vi "process_hit.vi"(7 "hammerIndex":i32, 11 "config":T1={"rate"=1652.0, "duration"=1.0, "thr"=100.0, "preTrigger"=100.0, "cutoff"=-3.0, "Filtro"=enum."Desativado", "highPass"=1000.0, "lowPass"=1000.0, "updateTime"=50.0} {"updateTime" format="%#_g ms"; "lowPass" format="%#_g Hz"; "highPass" format="%#_g Hz"; "cutoff" format="%#_g dB"; "preTrigger" format="%#_g ms"; "thr" format="%#_g N"; "duration" format="%#_g s"; "rate" min=1652.0 max=51200.0 format="%#_g Hz"}) -> ()   [LabVIEW 2016]
uses:
  MainFGV/Settings/Advanced/AdvancedConfig.ctl
  MainFGV/MainFGV_mods.ctl
panel:
  out "error out":errorcluster
  in  "error in":errorcluster
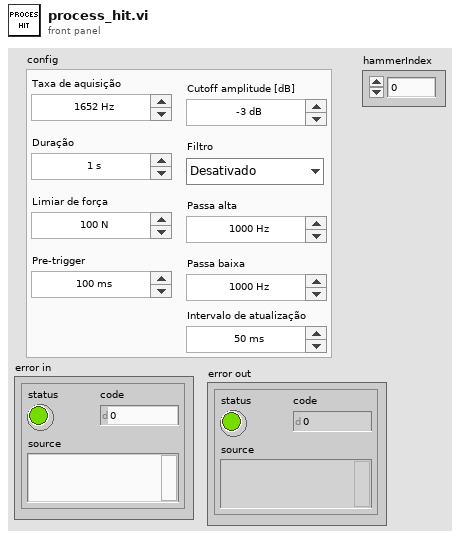
[diagram p1: front panel]
types:
  T1 = typedef "AdvancedConfig.ctl" = cluster{"rate":dbl, "duration":dbl, "thr":dbl, "preTrigger":dbl, "cutoff":dbl, "Filtro":enum16{"Desativado", "Passa banda", "Passa alta", "Passa baixa"}, "highPass":dbl, "lowPass":dbl, "updateTime":dbl}
  T2 = typedef "MainFGV_mods.ctl" = enum16{"Init", "Config", "Advanced", "CreateTask", "Register", "Start", "Record", "End"}
  T3 = typedef "results_data.ctl" = cluster{"config":T1, "hammer":waveform(dbl), "acelerometers":waveform(dbl)[], "hammerIndex":i32}
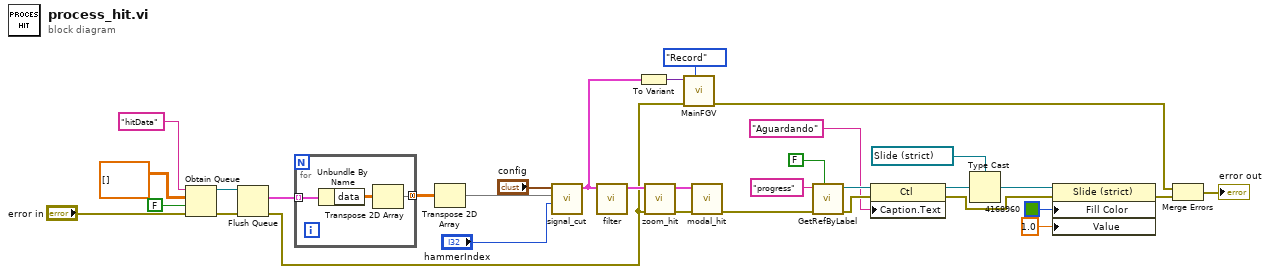
[diagram p0: block diagram]
diagram:
  n1 = Obtain Queue(name (unnamed)="hitData", element data type=dbl[][] [] ("data"), create if not found? (T)=FALSE, error in (no error)="error in") -> (queue out=w10:refnum<queue>, error out=w11:errorcluster)  [unwired: 1 in, 1 out]
  n2 = Flush Queue(queue=w10, error in (no error)=w11) -> (remaining elements=w9:cluster{"data":dbl[][]}[], error out=w5:errorcluster)  [unwired: 1 out]
  n3 = for {
    tunnel: w9 -> [w36] mode=indexing
    tunnel: [w34] -> w8 mode=concatenating
    n4 = Unbundle By Name(w36) -> ("data"=w35:dbl[][])
    n5 = Transpose 2D Array(2D array=w35) -> (transposed array=w34:dbl[][])
  }
  n6 = Transpose 2D Array(2D array=w8) -> (transposed array=w29:dbl[][])
  n7 = call "signal_cut.vi"("hammerIndex"="hammerIndex", "data"=w29, "config"="config") -> ("data_out"=w6:T3)  [unwired: 8 in]
  n8 = call "filter.vi"("data_in"=w6) -> ("data_out"=w30:T3)  [unwired: 10 in]
  n9 = To Variant(anything=w6) -> (Variant=w4:variant)
  n10 = call "zoom_hit.vi"("error in"=w5, "data_in"=w30) -> ("error out"=w17:errorcluster, "data_out"=w16:T3)  [unwired: 8 in]
  n11 = call "MainFGV.vi"("FGV_mods"=MainFGV_mods."Record", "Error In"=w5, "DataIn"=w4) -> ("Error Out"=w2:errorcluster)  [unwired: 7 in, 1 out]
  n12 = call "modal_hit.vi"("error in"=w17, "data_in"=w16) -> ("error out"=w15:errorcluster)  [unwired: 8 in, 1 out]
  n13 = call "GetRefByLabel.vi"("InsideTab"=FALSE, "error in"=w15, "Label"="progress") -> ("error out"=w27:errorcluster, "Ctl Refnum"=w26:refnum<vi>)  [unwired: 6 in, 1 out]
  n14 = property class="Ctl"(reference=w26, error in=w27, "Caption.Text"="Aguardando") -> (reference out=w23:refnum<vi>, error out=w21:errorcluster)
  n15 = Type Cast(type=refnum<vi> refnum ("progress"), x=w23) -> (*(type *) &x=w22:refnum<vi>)
  n16 = property class="Slide (strict)"(reference=w22, error in=w21, "Fill Color"=u32 4168960, "Value"=1.0) -> (error out=w3:errorcluster)  [unwired: 1 out]
  n17 = Merge Errors(w2, w3) -> (→"error out":errorcluster)
